vi "Actor Core.vi"(8 "error in":errorcluster, 11 "SingleIndi in":refnum<class "SingleIndi.lvclass">) -> (0 "error out":errorcluster, 3 "Actor out":refnum<class "Actor.lvclass">)   [LabVIEW 2020, in "SingleIndi.lvlib" / "SingleIndi.lvclass"]
doc: "(<B>Filename</B>: Actor Framework.lvlib:Actor.lvclass:Actor Core.vi)\n\nReceives messages to the actor, reacts to them, and initiates any error handling that may shut the actor down.\n\nDescendant classes may override this VI to append parallel tasks for the actor to complete while it handles messages. Overrides use the Call Parent Method node."
uses:
  SingleIndi.lvclass
  support/Actor Framework.lvlibp/1abvi3w/vi.lib/ActorFramework/Actor/Actor.lvclass
  SingleIndi.lvclass/SingleIndi.ctl
  D&C_SchemaBase/D&C_SchemaBase/D&C_SchemaBase.lvclass
panel:
  out "ChanVal":string
  in  "ChanSel":string(combo)
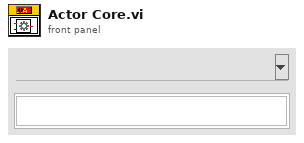
[diagram p1: front panel]
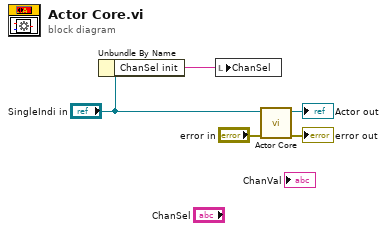
[diagram p0: block diagram]
diagram:
  n1 = Unbundle By Name("SingleIndi in") -> ("ChanSel init"=w1:string)
  n2 = local write "ChanSel"(w1) -> ()
  n3 = call-parent "Actor Core.vi"("error in"="error in", "UI_Actor in"="SingleIndi in") -> ("error out"=→"error out":errorcluster, "Actor out"=→"Actor out":refnum<class "Actor.lvclass">)  [unwired: 8 in]
